vi "FT10_Log Volt & Current TDMS Values.vi"(8 "error in (no error)":errorcluster, 9 "Log Cluster in":T2, 10 "Filename Cluster in":T1, 11 "Refnum in":T13) -> (0 "error out":errorcluster, 1 "Log Cluster out":T2, 2 "Filename Cluster out":T1, 3 "tdms file out":refnum<k34>)   [LabVIEW 2015]
uses:
  Controls/Control_Log TDMS Filename.ctl
  Controls/Control_Log Cluster.ctl
  Controls/Control_Log Time.ctl
  Controls/Control_Log Waveform Cluster - Current.ctl
  Controls/Control_Log Analysis Cluster - Current.ctl
  Controls/Control_Log Activation Settings Cluster.ctl
  Controls/Control_Log Unitherm Load.ctl
  Controls/Control_Log Port.ctl
  Controls/Control_Log Mode.ctl
  Controls/Control_Log Power Level.ctl
  Controls/Control_Log Waveform Cluster - Diff Voltage.ctl
  Controls/Control_Log Analysis Cluster - Diff Voltage.ctl
  Controls/Control_Log Filename Cluster.ctl
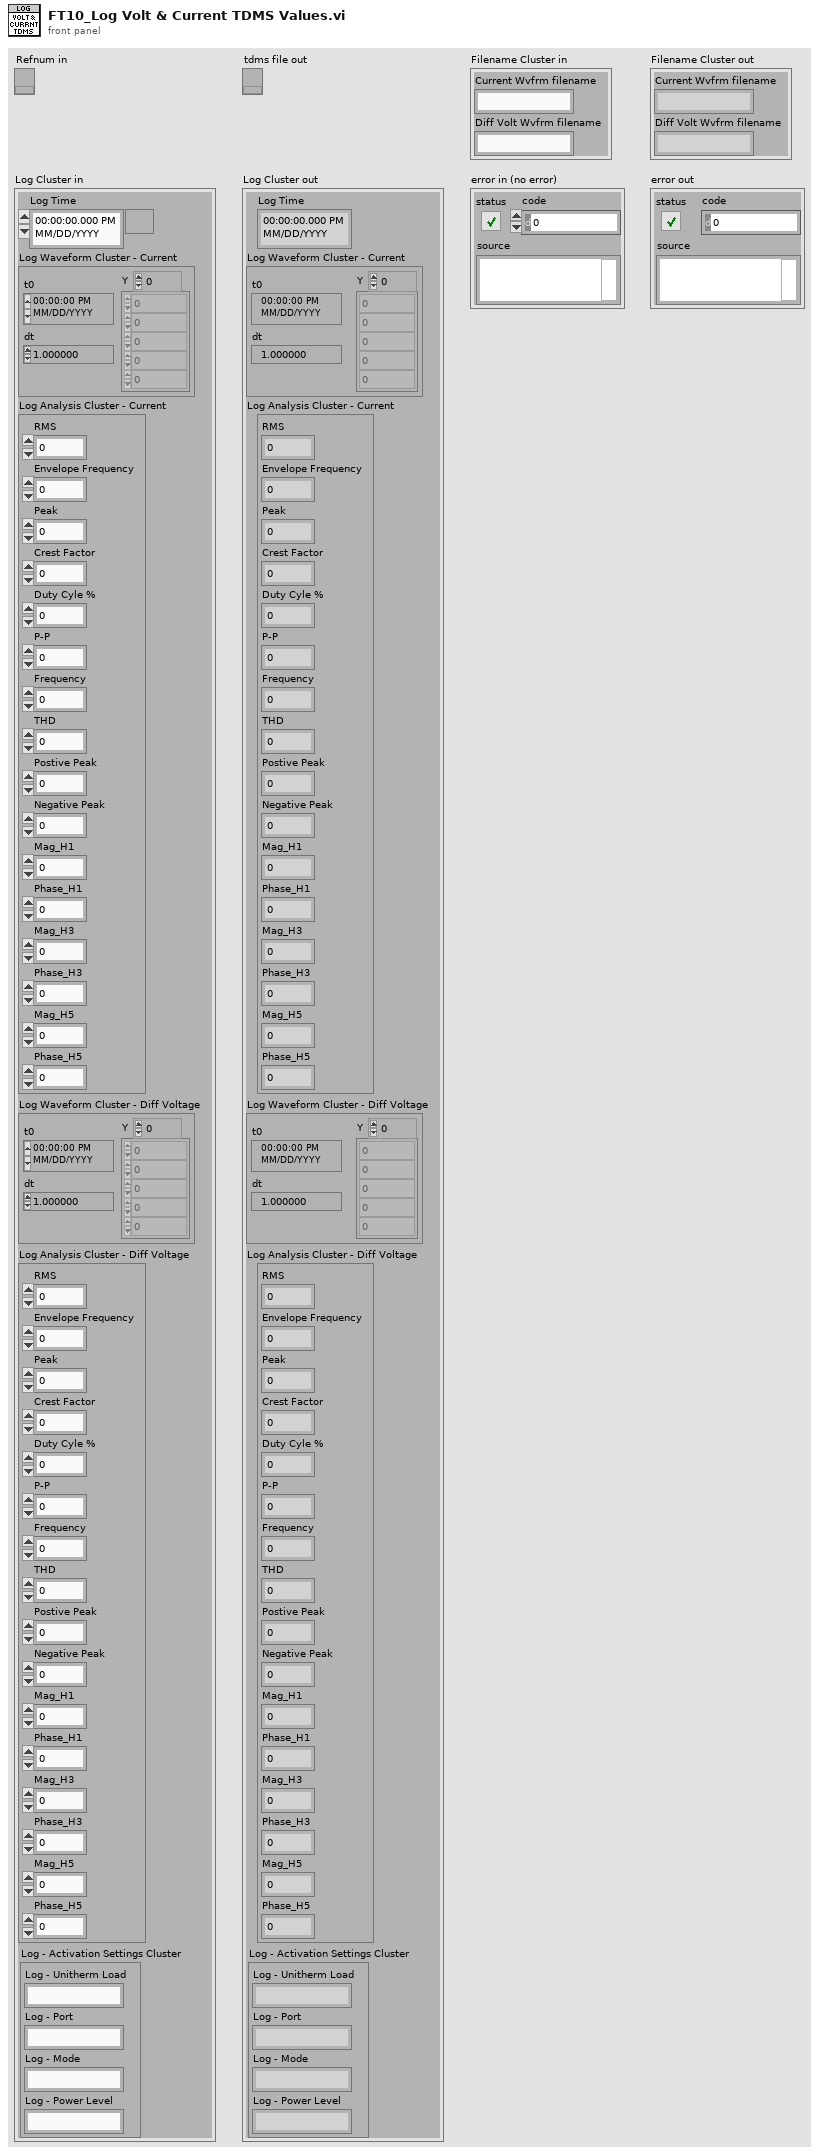
[diagram p1: front panel]
types:
  T1 = typedef "Control_Log Filename Cluster.ctl" = cluster{"Current Wvfrm filename":string, "Diff Volt Wvfrm filename":string}
  T2 = typedef "Control_Log Cluster.ctl" = cluster{"Log Time":T3, "Log Waveform Cluster - Current":T4, "Log Analysis Cluster - Current":T5, "Log - Activation Settings Cluster":T6, "Log Waveform Cluster - Diff Voltage":T11, "Log Analysis Cluster - Diff Voltage":T12}
  T3 = typedef "Control_Log Time.ctl" = timestamp
  T4 = typedef "Control_Log Waveform Cluster - Current.ctl" = waveform(dbl)
  T5 = typedef "Control_Log Analysis Cluster - Current.ctl" = cluster{"RMS":dbl, "Envelope Frequency":dbl, "Peak":dbl, "Crest Factor":dbl, "Duty Cyle %":dbl, "P-P":dbl, "Frequency":dbl, "THD":dbl, "Postive Peak":dbl, "Negative Peak":dbl, "Mag_H1":dbl, "Phase_H1":dbl, "Mag_H3":dbl, "Phase_H3":dbl, "Mag_H5":dbl, "Phase_H5":dbl}
  T6 = typedef "Control_Log Activation Settings Cluster.ctl" = cluster{"Log - Unitherm Load":T7, "Log - Port":T8, "Log - Mode":T9, "Log - Power Level":T10}
  T7 = typedef "Control_Log Unitherm Load.ctl" = string
  T8 = typedef "Control_Log Port.ctl" = string
  T9 = typedef "Control_Log Mode.ctl" = string
  T10 = typedef "Control_Log Power Level.ctl" = string
  T11 = typedef "Control_Log Waveform Cluster - Diff Voltage.ctl" = waveform(dbl)
  T12 = typedef "Control_Log Analysis Cluster - Diff Voltage.ctl" = cluster{"RMS":dbl, "Envelope Frequency":dbl, "Peak":dbl, "Crest Factor":dbl, "Duty Cyle %":dbl, "P-P":dbl, "Frequency":dbl, "THD":dbl, "Postive Peak":dbl, "Negative Peak":dbl, "Mag_H1":dbl, "Phase_H1":dbl, "Mag_H3":dbl, "Phase_H3":dbl, "Mag_H5":dbl, "Phase_H5":dbl}
  T13 = typedef "Control_Log TDMS Filename.ctl" = refnum<k34>
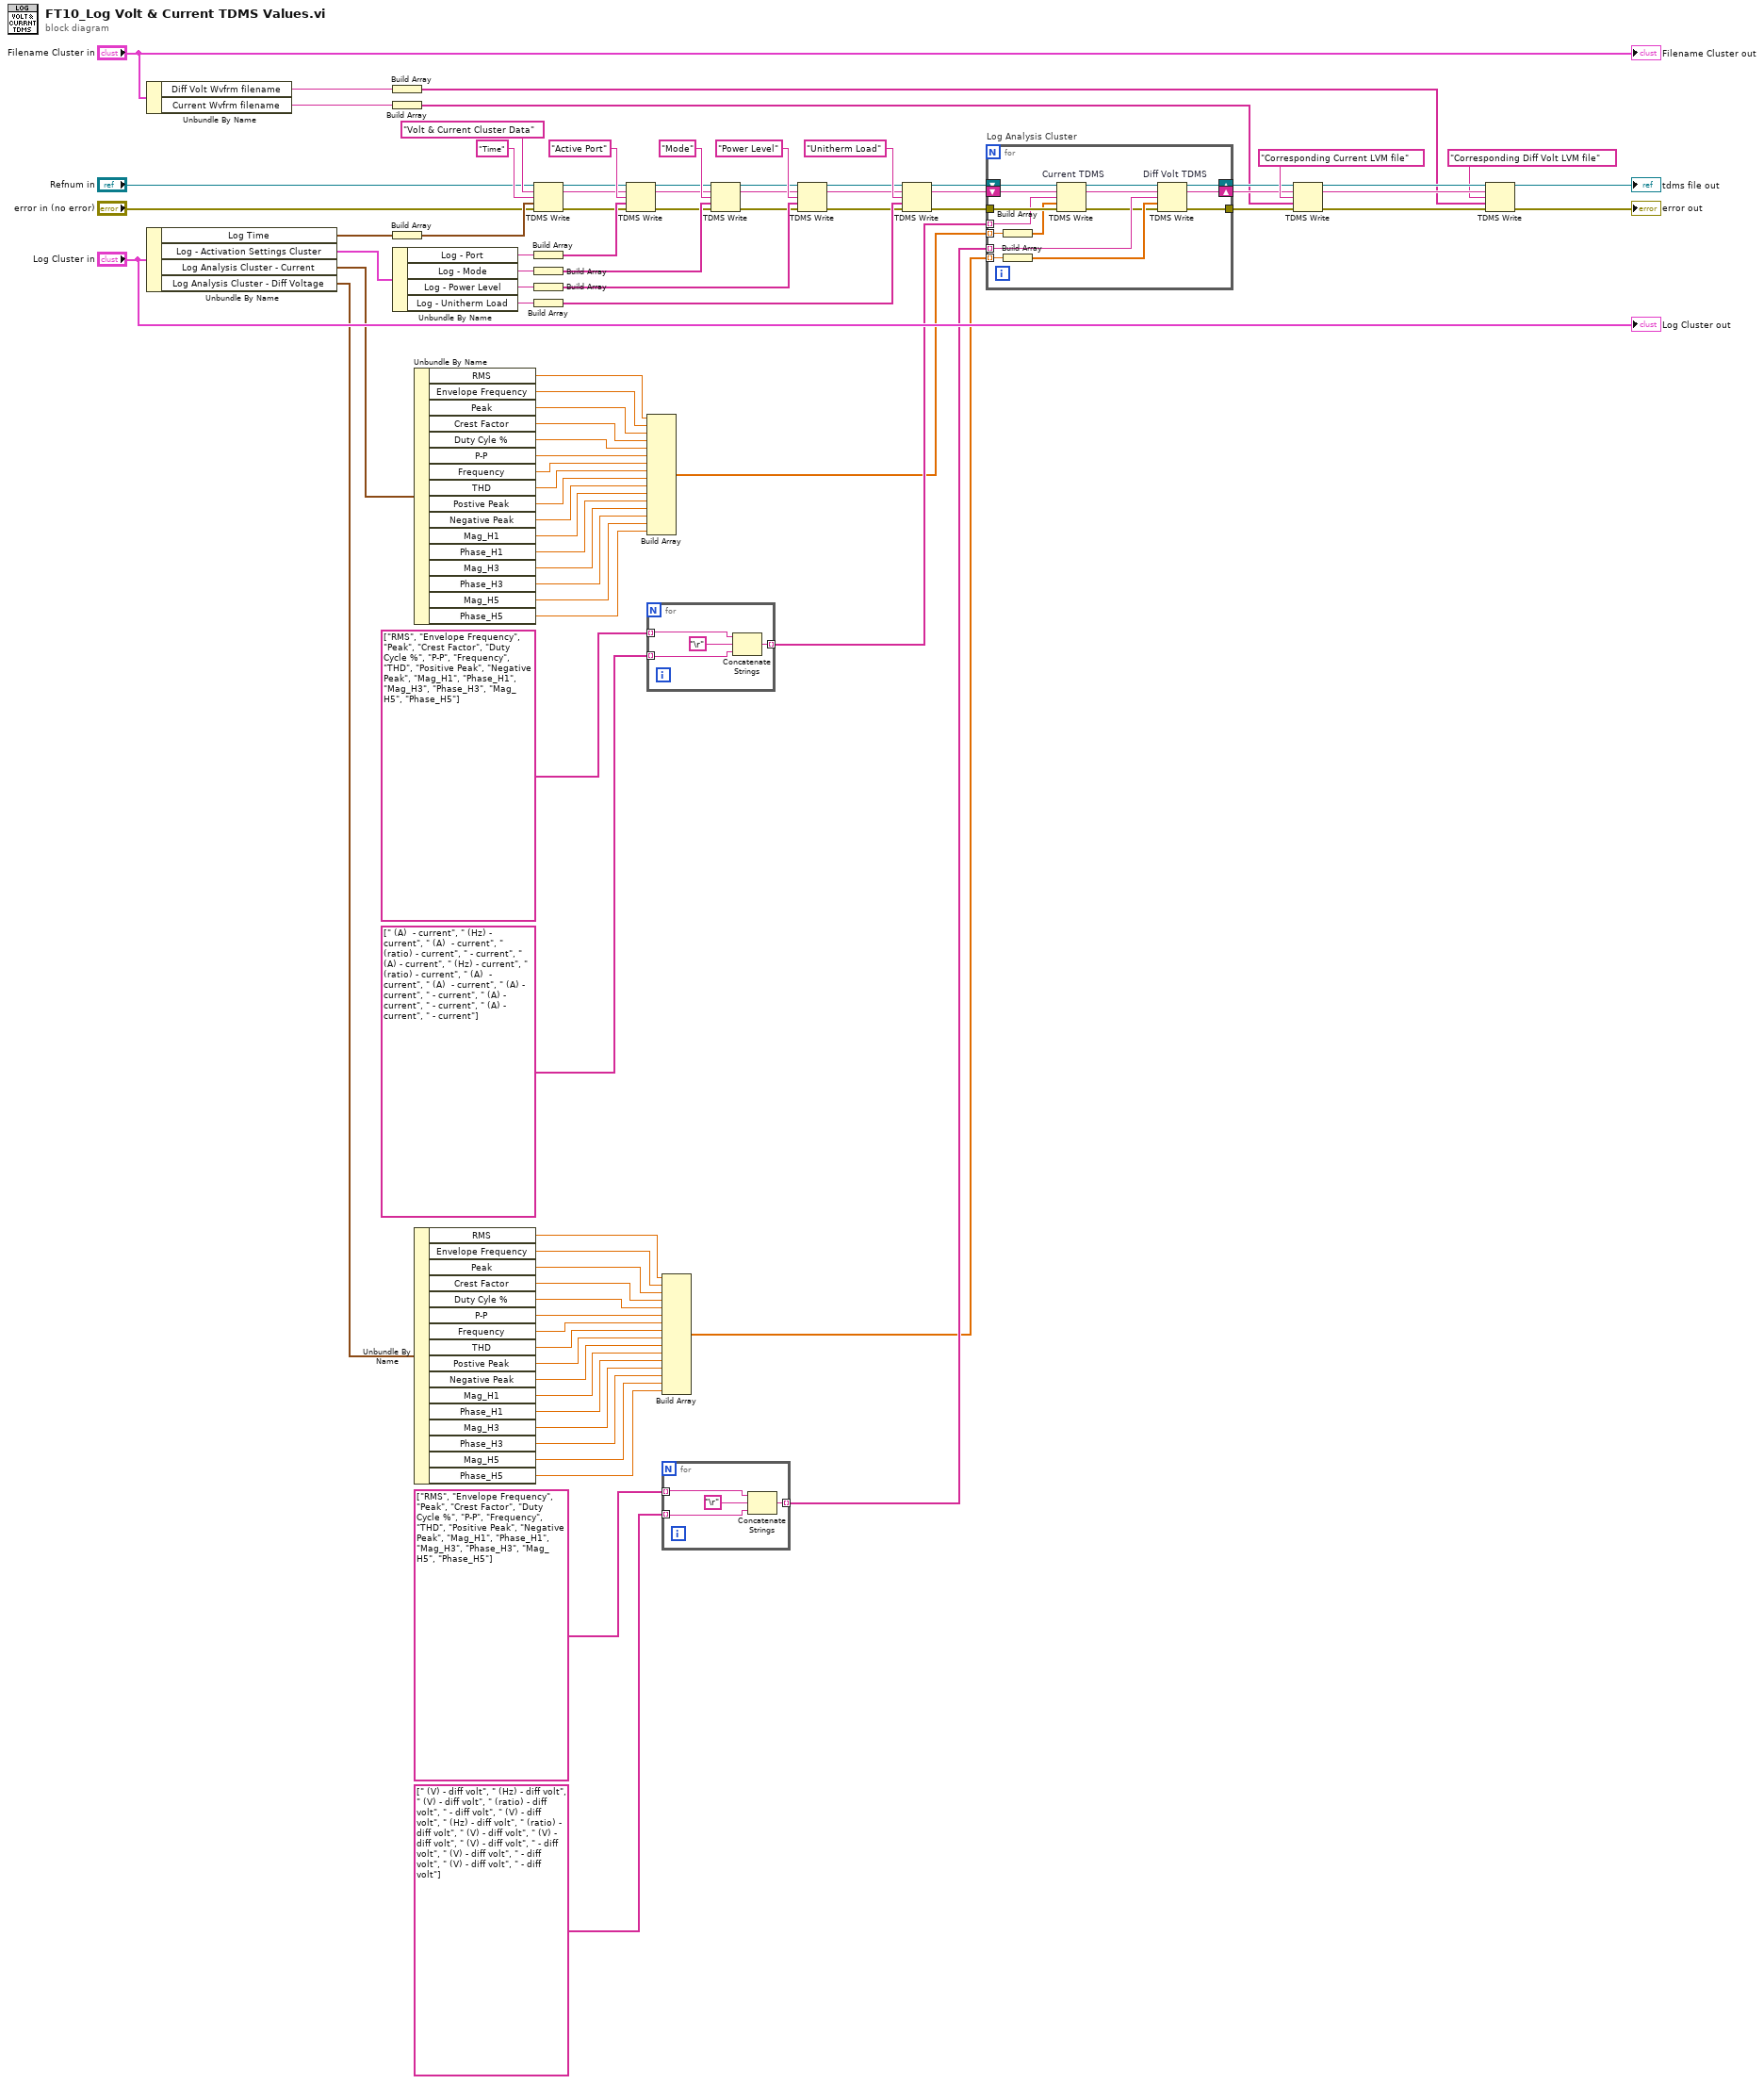
[diagram p0: block diagram]
diagram:
  n1 = Unbundle By Name("Filename Cluster in") -> ("Diff Volt Wvfrm filename"=w41:string, "Current Wvfrm filename"=w46:string)
  n2 = Unbundle By Name("Log Cluster in") -> ("Log Time"=w52:T3, "Log - Activation Settings Cluster"=w43:T6, "Log Analysis Cluster - Current"=w42:T5, "Log Analysis Cluster - Diff Voltage"=w15:T12)
  n3 = Build Array(w41) -> (w35:string[])
  n4 = Build Array(w46) -> (w44:string[])
  n5 = Build Array(w52) -> (w53:T3[])
  n6 = Unbundle By Name(w43) -> ("Log - Port"=w85:T8, "Log - Mode"=w87:T9, "Log - Power Level"=w89:T10, "Log - Unitherm Load"=w10:T7)
  n7 = Unbundle By Name(w42) -> ("RMS"=w56:dbl, "Envelope Frequency"=w57:dbl, "Peak"=w58:dbl, "Crest Factor"=w59:dbl, "Duty Cyle %"=w60:dbl, "P-P"=w61:dbl, "Frequency"=w62:dbl, "THD"=w63:dbl, "Postive Peak"=w64:dbl, "Negative Peak"=w65:dbl, "Mag_H1"=w66:dbl, "Phase_H1"=w67:dbl, "Mag_H3"=w68:dbl, "Phase_H3"=w69:dbl, "Mag_H5"=w70:dbl, "Phase_H5"=w71:dbl)
  n8 = Unbundle By Name(w15) -> ("RMS"=w18:dbl, "Envelope Frequency"=w19:dbl, "Peak"=w20:dbl, "Crest Factor"=w21:dbl, "Duty Cyle %"=w22:dbl, "P-P"=w23:dbl, "Frequency"=w24:dbl, "THD"=w25:dbl, "Postive Peak"=w26:dbl, "Negative Peak"=w27:dbl, "Mag_H1"=w28:dbl, "Phase_H1"=w29:dbl, "Mag_H3"=w30:dbl, "Phase_H3"=w31:dbl, "Mag_H5"=w32:dbl, "Phase_H5"=w33:dbl)
  n9 = TDMS Write(0:"Refnum in", 5:"Volt & Current Cluster Data" ("group name in (Untitled)"), 7:"Time" ("channel name(s) in (Untitled)"), 9:w53, 11:"error in (no error)") -> (4:w80:refnum<k34>, 6:w78:string, 15:w83:errorcluster)  [unwired: 1 in, 1 out]
  n10 = Build Array(w85) -> (w86:T8[])
  n11 = Build Array(w87) -> (w88:T9[])
  n12 = Build Array(w89) -> (w7:T10[])
  n13 = Build Array(w10) -> (w8:T7[])
  n14 = TDMS Write(0:w80, 5:w78, 7:"Active Port" ("channel name(s) in (Untitled)"), 9:w86, 11:w83) -> (4:w81:refnum<k34>, 6:w77:string, 15:w84:errorcluster)  [unwired: 1 in, 1 out]
  n15 = Build Array(w56, w57, w58, w59, w60, w61, w62, w63, w64, w65, w66, w67, w68, w69, w70, w71) -> (w12:dbl[])
  n16 = for {
    tunnel: string[] ["RMS", "Envelope Frequency", "Peak", "Crest Factor", "Duty Cycle %", "P-P", "Frequency", "THD", "Positive Peak", "Negative Peak", "Mag_H1", "Phase_H1", "Mag_H3", "Phase_H3", "Mag_H5", "Phase_H5"] ("channel name(s) in (Untitled)") -> [w95] mode=indexing
    tunnel: string[] [" (A)  - current", " (Hz) - current", " (A)  - current", " (ratio) - current", " - current", " (A) - current", " (Hz) - current", " (ratio) - current", " (A)  - current", " (A)  - current", " (A) - current", " - current", " (A) - current", " - current", " (A) - current", " - current"] ("channel name(s) in (Untitled)") -> [w94] mode=indexing
    tunnel: [w93] -> w14 mode=indexing
    n17 = Concatenate Strings(w95, "\r", w94) -> (w93:string)
  }
  n18 = Build Array(w18, w19, w20, w21, w22, w23, w24, w25, w26, w27, w28, w29, w30, w31, w32, w33) -> (w11:dbl[])
  n19 = for {
    tunnel: string[] ["RMS", "Envelope Frequency", "Peak", "Crest Factor", "Duty Cycle %", "P-P", "Frequency", "THD", "Positive Peak", "Negative Peak", "Mag_H1", "Phase_H1", "Mag_H3", "Phase_H3", "Mag_H5", "Phase_H5"] ("channel name(s) in (Untitled)") -> [w99] mode=indexing
    tunnel: string[] [" (V) - diff volt", " (Hz) - diff volt", " (V) - diff volt", " (ratio) - diff volt", " - diff volt", " (V) - diff volt", " (Hz) - diff volt", " (ratio) - diff volt", " (V) - diff volt", " (V) - diff volt", " (V) - diff volt", " - diff volt", " (V) - diff volt", " - diff volt", " (V) - diff volt", " - diff volt"] ("channel name(s) in (Untitled)") -> [w98] mode=indexing
    tunnel: [w97] -> w13 mode=indexing
    n20 = Concatenate Strings(w99, "\r", w98) -> (w97:string)
  }
  n21 = TDMS Write(0:w81, 5:w77, 7:"Mode" ("channel name(s) in (Untitled)"), 9:w88, 11:w84) -> (4:w6:refnum<k34>, 6:w5:string, 15:w4:errorcluster)  [unwired: 1 in, 1 out]
  n22 = TDMS Write(0:w6, 5:w5, 7:"Power Level" ("channel name(s) in (Untitled)"), 9:w7, 11:w4) -> (4:w3:refnum<k34>, 6:w2:string, 15:w1:errorcluster)  [unwired: 1 in, 1 out]
  n23 = TDMS Write(0:w3, 5:w2, 7:"Unitherm Load" ("channel name(s) in (Untitled)"), 9:w8, 11:w1) -> (4:w79:refnum<k34>, 6:w76:string, 15:w82:errorcluster)  [unwired: 1 in, 1 out]
  n24 = for "Log Analysis Cluster" {
    shift-right: [w106] -> w73
    shift-left: w79 -> [w115]
    shift-right: [w105] -> w74
    shift-left: w76 -> [w114]
    tunnel: w82 -> [w113]
    tunnel: [w104] -> w72
    tunnel: w12 -> [w112] mode=indexing
    tunnel: w14 -> [w110] mode=indexing
    tunnel: w13 -> [w108] mode=indexing
    tunnel: w11 -> [w107] mode=indexing
    n25 = Build Array(w112) -> (w111:dbl[])
    n26 = Build Array(w107) -> (w109:dbl[])
    n27 = TDMS Write "Current TDMS"(0:w115, 5:w114, 7:w110, 9:w111, 11:w113) -> (4:w103:refnum<k34>, 6:w102:string, 15:w101:errorcluster)  [unwired: 1 in, 1 out]
    n28 = TDMS Write "Diff Volt TDMS"(0:w103, 5:w102, 7:w108, 9:w109, 11:w101) -> (4:w106:refnum<k34>, 6:w105:string, 15:w104:errorcluster)  [unwired: 1 in, 1 out]
  }
  n29 = TDMS Write(0:w73, 5:w74, 7:"Corresponding Current LVM file" ("channel name(s) in (Untitled)"), 9:w44, 11:w72) -> (4:w40:refnum<k34>, 6:w36:string, 15:w38:errorcluster)  [unwired: 1 in, 1 out]
  n30 = TDMS Write(0:w40, 5:w36, 7:"Corresponding Diff Volt LVM file" ("channel name(s) in (Untitled)"), 9:w35, 11:w38) -> (4:→"tdms file out":refnum<k34>, 15:→"error out":errorcluster)  [unwired: 1 in, 2 out]
  "Log Cluster out" <- "Log Cluster in"
  "Filename Cluster out" <- "Filename Cluster in"
